vi "Configure Function.vi"(0 "VISA Resource Name":refnum<visa-resource-name>, 1 "function range (None)":dbl caption="Function Range (0 (None))" format="%^.2e", 5 "Source (\"Channel 1\")":string(combo)="CHAN1", 7 "operation (Subtract)":i32(ring) caption="Operation (0: Subtract)" items=["Subtract", "Multiply", "FFT", "Differentiate", "Integrate"], 9 "function enabled (False)":bool caption="Function Enabled (False)", 11 "error in (no error)":errorcluster {"code" format="%.0x"}, 12 "function offset (None)":dbl caption="Function Offset (0 (None))" format="%^.2e") -> (4 "VISA Resource Name Out":refnum<visa-resource-name>, 15 "error out":errorcluster {"code" format="%.0x"})   [LabVIEW 2011, in "Agilent 546XX Series.lvlib"]
doc: "This VI configures the function operation, function source, function enabled, function range and offset."
uses:
  Agilent 546XX Series.lvlib
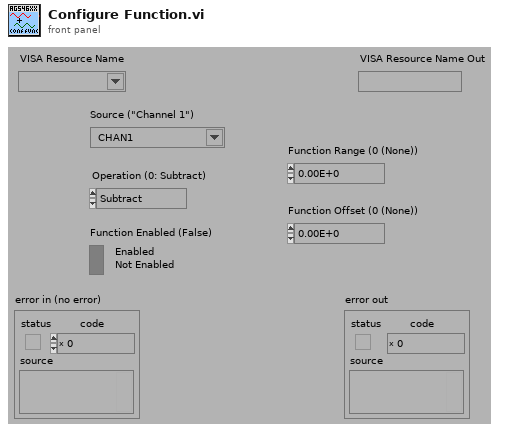
[diagram p1: front panel]
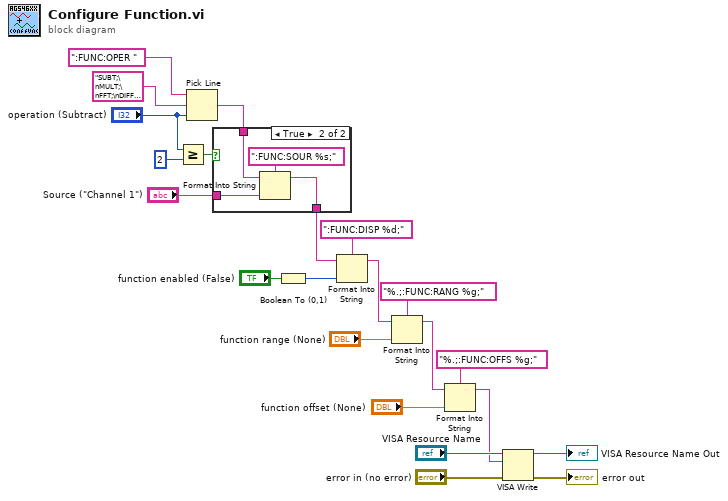
[diagram p0: block diagram]
diagram:
  n1 = Greater Or Equal?(x="operation (Subtract)", y=2) -> (x >= y?=w16:bool)
  n2 = Pick Line(string ("")=":FUNC:OPER ", multi-line string="SUBT;\nMULT;\nFFT;\nDIFF;\nINT;", line index="operation (Subtract)") -> (output string=w12:string)
  n3 = case shown="True" w16 {
    tunnel: "Source (\"Channel 1\")" -> [_ w27]
    tunnel: w12 -> [w23 w26]
    tunnel: [w23 w24] -> w8
    frame False {
    }
    frame True {
      n4 = Format Into String(format string=":FUNC:SOUR %s;", initial string=w26, w27) -> (resulting string=w24:string)  [unwired: 1 in, 1 out]
    }
  }
  n5 = Boolean To (0,1)(Boolean="function enabled (False)") -> (0, 1=w10:i16)
  n6 = Format Into String(format string=":FUNC:DISP %d;", initial string=w8, w10) -> (resulting string=w5:string)  [unwired: 1 in, 1 out]
  n7 = Format Into String(format string="%.;:FUNC:RANG %g;", initial string=w5, "function range (None)") -> (resulting string=w4:string)  [unwired: 1 in, 1 out]
  n8 = Format Into String(format string="%.;:FUNC:OFFS %g;", initial string=w4, "function offset (None)") -> (resulting string=w1:string)  [unwired: 1 in, 1 out]
  n9 = VISA Write(VISA resource name="VISA Resource Name", write buffer=w1, error in (no error)="error in (no error)") -> (VISA resource name out=→"VISA Resource Name Out":refnum<visa-resource-name>, error out=→"error out":errorcluster)  [unwired: 1 out]
